vi "pf_Parse_StatusLine.vi"(11 "Status Line":u8[][](array[numeric])) -> (0 "MissedTriggerCounter":u8[](array[numeric]), 1 "EncoderPosition":u32[](array[numeric]), 2 "RealTimeCounter":u32[](array[numeric]), 3 "ImageCounter":u32[](array[numeric]), 4 "MissedBurstTriggerCounter":u8[](array[numeric]), 6 "MissedFrameCombineTriggerCounter":u8[](array[numeric]))   [LabVIEW 2025, in "Photonfocus_Toolkit.lvlib"]
uses:
  Photonfocus_Toolkit.lvlib
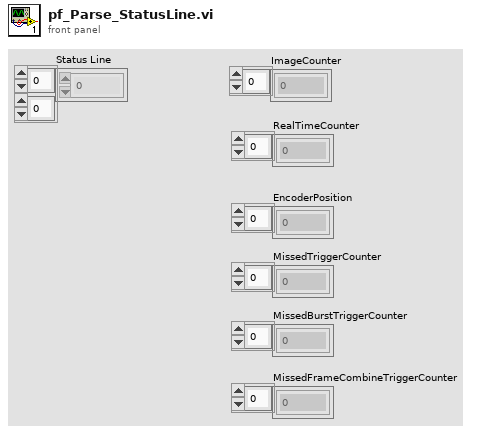
[diagram p1: front panel]
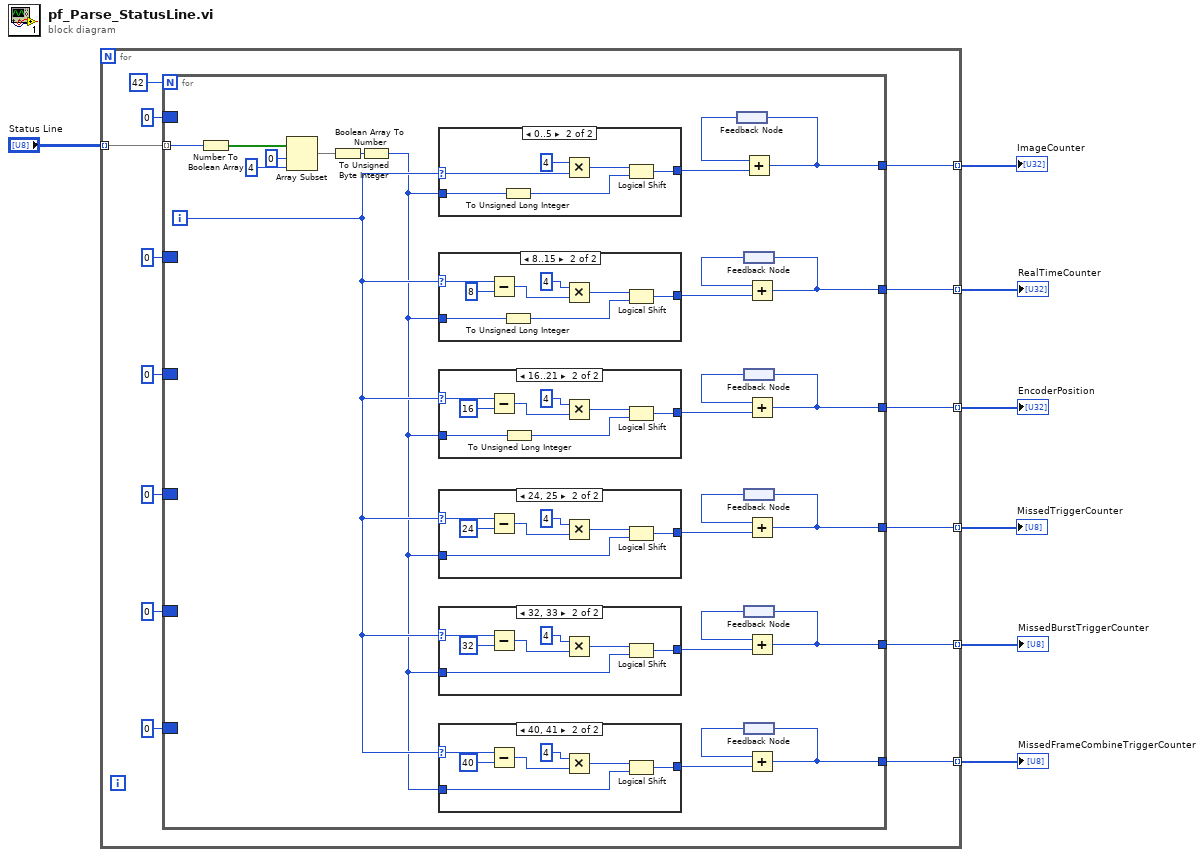
[diagram p0: block diagram]
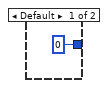
[diagram p2: hidden frame]
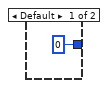
[diagram p3: hidden frame]
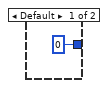
[diagram p4: hidden frame]
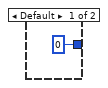
[diagram p5: hidden frame]
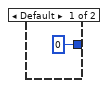
[diagram p6: hidden frame]
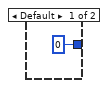
[diagram p7: hidden frame]
diagram:
  n1 = for {
    tunnel: "Status Line" -> [w21] mode=indexing
    tunnel: [w19] -> w6 mode=indexing
    tunnel: [w16] -> w5 mode=indexing
    tunnel: [w14] -> w4 mode=indexing
    tunnel: [w11] -> w3 mode=indexing
    tunnel: [w10] -> w2 mode=indexing
    tunnel: [w8] -> w1 mode=indexing
    n2 = for {
      N: 42 -> [_]
      tunnel: w21 -> [w41] mode=indexing
      tunnel: [w40] -> w19
      border: u32 0 -> [_]
      border: u32 0 -> [_]
      tunnel: [w37] -> w16
      border: u32 0 -> [_]
      tunnel: [w34] -> w14
      border: u8 0 -> [_]
      border: u8 0 -> [_]
      tunnel: [w28] -> w11
      tunnel: [w27] -> w10
      border: u8 0 -> [_]
      tunnel: [w22] -> w8
      i -> [w24]
      n3 = Number To Boolean Array(number=w41) -> (Boolean array=w45:bool[])
      n4 = Array Subset(array=w45, index=0, length=4) -> (w43:bool[])
      n5 = Boolean Array To Number(Boolean array=w43) -> (number=w44:u32)
      n6 = To Unsigned Byte Integer(number=w44) -> (unsigned 8bit integer=w23:u8)
      n7 = case shown="0..5" w24 {
        selector: w24 -> [_ w74]
        tunnel: [u32 0 w75] -> w33
        tunnel: w23 -> [_ w76]
        frame Default {
        }
        frame 0..5 {
          n8 = To Unsigned Long Integer(number=w76) -> (unsigned 32bit integer=w73:u32)
          n9 = Multiply(x=4, y=w74) -> (x*y=w78:i32)
          n10 = Logical Shift(y=w78, x=w73) -> (x << y=w75:u32)
        }
      }
      n11 = case shown="8..15" w24 {
        selector: w24 -> [_ w94]
        tunnel: [u32 0 w90] -> w38
        tunnel: w23 -> [_ w91]
        frame Default {
        }
        frame 8..15 {
          n12 = Subtract(x=w94, y=8) -> (x-y=w92:i32)
          n13 = To Unsigned Long Integer(number=w91) -> (unsigned 32bit integer=w89:u32)
          n14 = Multiply(x=4, y=w92) -> (x*y=w96:i32)
          n15 = Logical Shift(y=w96, x=w89) -> (x << y=w90:u32)
        }
      }
      n16 = case shown="16..21" w24 {
        selector: w24 -> [_ w85]
        tunnel: [u32 0 w81] -> w35
        tunnel: w23 -> [_ w82]
        frame Default {
        }
        frame 16..21 {
          n17 = Subtract(x=w85, y=16) -> (x-y=w83:i32)
          n18 = To Unsigned Long Integer(number=w82) -> (unsigned 32bit integer=w80:u32)
          n19 = Multiply(x=4, y=w83) -> (x*y=w87:i32)
          n20 = Logical Shift(y=w87, x=w80) -> (x << y=w81:u32)
        }
      }
      n21 = case shown="24, 25" w24 {
        selector: w24 -> [_ w69]
        tunnel: [u8 0 w65] -> w31
        tunnel: w23 -> [_ w66]
        frame Default {
        }
        frame 24, 25 {
          n22 = Subtract(x=w69, y=24) -> (x-y=w67:i32)
          n23 = Multiply(x=4, y=w67) -> (x*y=w71:i32)
          n24 = Logical Shift(y=w71, x=w66) -> (x << y=w65:u8)
        }
      }
      n25 = case shown="32, 33" w24 {
        selector: w24 -> [_ w61]
        tunnel: [u8 0 w57] -> w29
        tunnel: w23 -> [_ w58]
        frame Default {
        }
        frame 32, 33 {
          n26 = Subtract(x=w61, y=32) -> (x-y=w59:i32)
          n27 = Multiply(x=4, y=w59) -> (x*y=w63:i32)
          n28 = Logical Shift(y=w63, x=w58) -> (x << y=w57:u8)
        }
      }
      n29 = case shown="40, 41" w24 {
        selector: w24 -> [_ w53]
        tunnel: [u8 0 w49] -> w25
        tunnel: w23 -> [_ w50]
        frame Default {
        }
        frame 40, 41 {
          n30 = Subtract(x=w53, y=40) -> (x-y=w51:i32)
          n31 = Multiply(x=4, y=w51) -> (x*y=w55:i32)
          n32 = Logical Shift(y=w55, x=w50) -> (x << y=w49:u8)
        }
      }
      n33 = feedback #1() -> (w42:u32)
      n34 = Add(x=w42, y=w33) -> (x+y=w40:u32)
      n35 = feedback-in #1(w40) -> ()
      n36 = feedback #2() -> (w39:u32)
      n37 = feedback #3() -> (w36:u32)
      n38 = feedback #4() -> (w32:u8)
      n39 = feedback #5() -> (w30:u8)
      n40 = feedback #6() -> (w26:u8)
      n41 = Add(x=w39, y=w38) -> (x+y=w37:u32)
      n42 = feedback-in #2(w37) -> ()
      n43 = Add(x=w36, y=w35) -> (x+y=w34:u32)
      n44 = feedback-in #3(w34) -> ()
      n45 = Add(x=w32, y=w31) -> (x+y=w28:u8)
      n46 = feedback-in #4(w28) -> ()
      n47 = Add(x=w30, y=w29) -> (x+y=w27:u8)
      n48 = feedback-in #5(w27) -> ()
      n49 = Add(x=w26, y=w25) -> (x+y=w22:u8)
      n50 = feedback-in #6(w22) -> ()
    }
  }
  "ImageCounter" <- w6
  "RealTimeCounter" <- w5
  "EncoderPosition" <- w4
  "MissedTriggerCounter" <- w3
  "MissedBurstTriggerCounter" <- w2
  "MissedFrameCombineTriggerCounter" <- w1
